vi "BRig_Host_dataRunState_dataPlot_DAB_flipLR.vi"() -> (2 "output_idx_dataPlot_DAB_flipLR":i32)   [LabVIEW 2014]
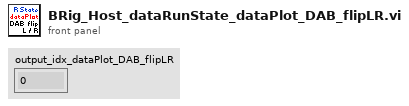
[diagram p1: front panel]
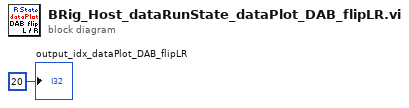
[diagram p0: block diagram]
diagram:
  "output_idx_dataPlot_DAB_flipLR" <- 20 ("output_idx_dataTS")
